vi "PID_controller_02.vi"() -> ()   [LabVIEW 2011]
uses:
  <vilib>/Platform/TimedLoop/XDataNode/nitl_modes.ctl
  <vilib>/Platform/TimedLoop/XDataNode/timing_clust.ctl
  <vilib>/Platform/TimedLoop/XDataNode/wakeup.ctl
  <vilib>/Platform/TimedLoop/XDataNode/XDataNode.xnode
  <vilib>/Platform/TimedLoop/XDataNode/XDNodeRunTimeDep.lvlib
panel:
  out "tan(angle)":dbl
  in  "stop":bool
  out "duration (s)":dbl
  in  "Period (s)":dbl
  out "Process value":dbl
  out "prev error":dbl
  out "derivative":dbl
  out "integral":dbl
  out "error":dbl
  out "Current angle (deg)":dbl
  in  "Kd":dbl
  in  "Ki":dbl
  in  "Kp":dbl
  out "Current value (torr)":dbl
  in  "Set Point (torr)":dbl
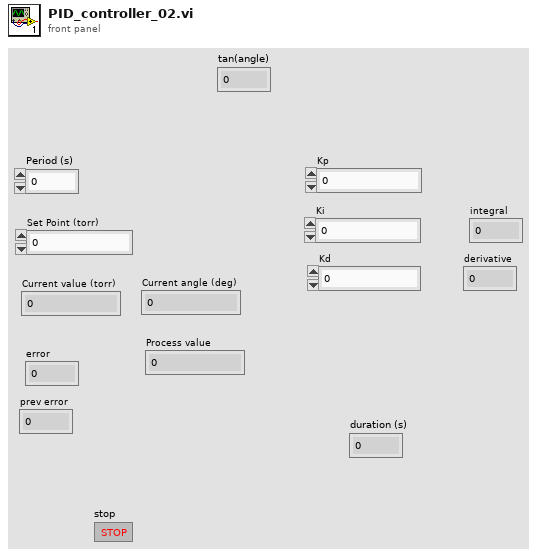
[diagram p1: front panel]
types:
  T1 = typedef "XDNodeRunTimeDep.lvlib/nitl_modes.ctl" = enum32{"No Change", "Process missed periods, maintain original phase", "Discard missed periods, maintain original phase", "Process missed periods, ignore original phase", "Discard missed periods, ignore original phase"}
  T2 = typedef "XDNodeRunTimeDep.lvlib/timing_clust.ctl" = cluster{"Expected End [f-1]":u64, "Actual End [f-1]":u64, "Finished Late? [f-1]":bool, "Expected End [i-1]":u64, "Actual End [i-1]":u64, "Finished Late? [i-1]":bool, "Expected Start [i]":u64, "Actual Start [i]":u64, "Expected Start [f]":u64, "Actual Start [f]":u64, "Source Name":string, "Structure Name":string, "Period":i64, "Deadline":i64, "Offset":i64, "Start":i64, "Priority":i32, "Timeout":i32, "Mode":T1, "Wakeup Reason":T3, "Error":errorcluster, "Source Type":string, "Secondary Source Type":string, "Global End Time":u64, "Global Start Time":u64, "Frame Duration":u64, "Iteration Duration":u64, "Assigned CPU":i32, "I/O Scan Engine Mode":u32}
  T3 = typedef "XDNodeRunTimeDep.lvlib/wakeup.ctl" = enum32{"Normal", "Aborted", "Asynchronous wakeup", "Timing source error", "Timed loop error", "Timeout"}
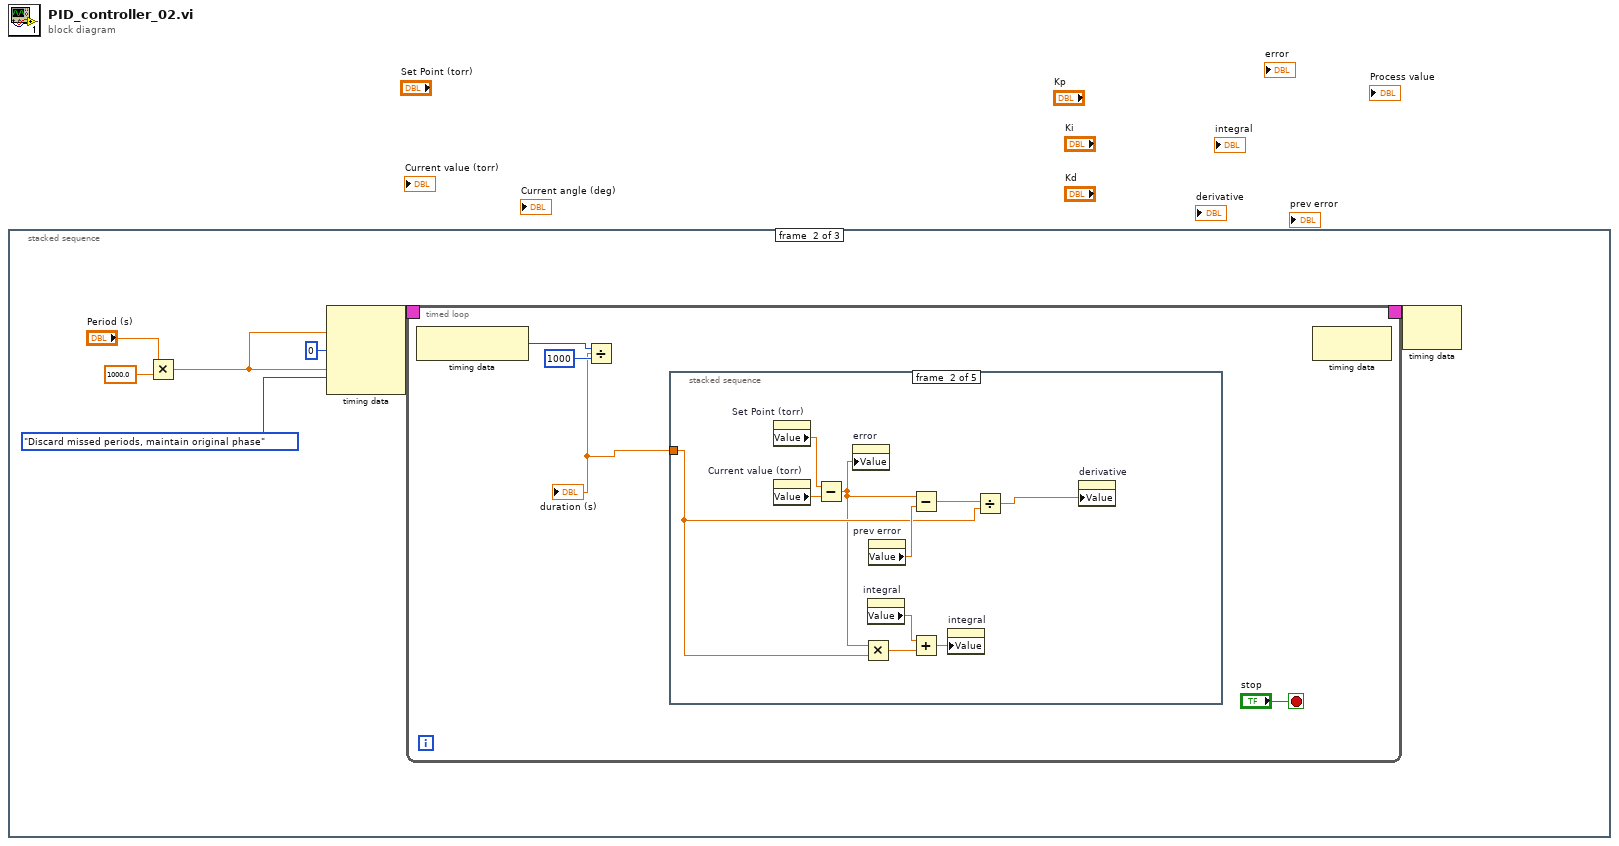
[diagram p0: block diagram]
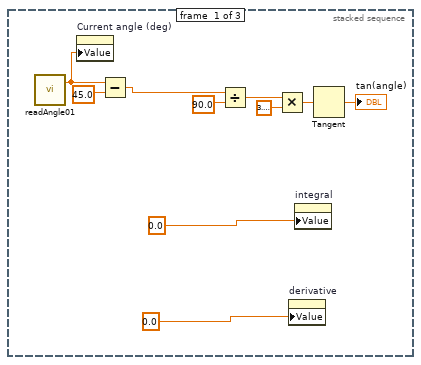
[diagram p2: hidden frame]
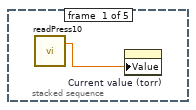
[diagram p3: hidden frame]
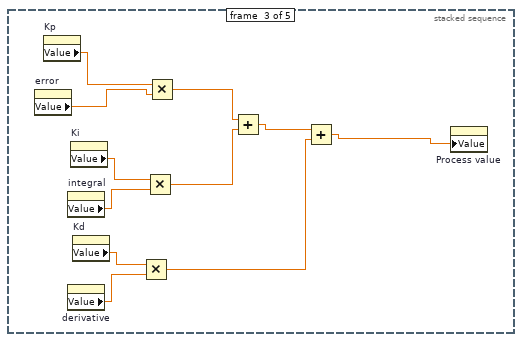
[diagram p4: hidden frame]
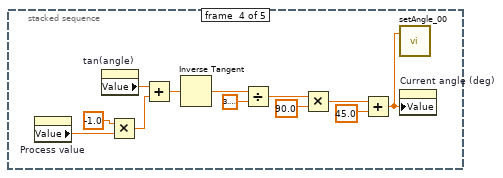
[diagram p5: hidden frame]
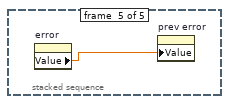
[diagram p6: hidden frame]
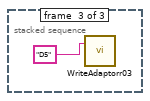
[diagram p7: hidden frame]
diagram:
  n1 = stacked-sequence {
    frame #0 {
      n2 = call "readAngle01.vi"() -> ("angle"=w7:dbl)  [unwired: 1 in, 1 out]
      n3 = property on="Current angle (deg)" class="DigNum (strict)"("Value"=w7) -> ()  [unwired: 2 in, 2 out]
      n4 = Subtract(x=w7, y=45.0) -> (x-y=w1:dbl)
      n5 = Divide(x=w1, y=90.0) -> (x/y=w5:dbl)
      n6 = Multiply(x=w5, y=3.141592653589793) -> (x*y=w3:dbl)
      n7 = property on="derivative" class="DigNum (strict)"("Value"=0.0 ("derivative")) -> ()  [unwired: 2 in, 2 out]
      n8 = property on="integral" class="DigNum (strict)"("Value"=0.0 ("integral")) -> ()  [unwired: 2 in, 2 out]
      n9 = Tangent(1:w3) -> (0:→"tan(angle)":dbl)
    }
    frame #1 {
      n10 = Multiply(x="Period (s)", y=1000.0) -> (x*y=w12:dbl)
      n11 = node-c288(w12, i64 0 ("Offset"), w12, nitl_modes."Discard missed periods, maintain original phase" ("Mode")) -> (w17:T2)
      n12 = timed-loop {
        timing: w17 -> [_]
        timing-out: [_] -> w16
        stop <- "stop" stop-if-true
        n13 = node-c288() -> (w21:i64)  [unwired: 1 in]
        n14 = Divide(x=w21, y=i64 1000) -> (x/y=w19:dbl)
        "duration (s)" <- w19
        n15 = stacked-sequence {
          tunnel: w19 -> [_ w26 _ _ _]
          frame #0 {
            n16 = call "readPress10.vi"() -> ("P"=w22:dbl)  [unwired: 1 in, 1 out]
            n17 = property on="Current value (torr)" class="DigNum (strict)"("Value"=w22) -> ()  [unwired: 2 in, 2 out]
          }
          frame #1 {
            n18 = property on="Set Point (torr)" class="DigNum (strict)"() -> ("Value"=w28:dbl)  [unwired: 2 in, 2 out]
            n19 = property on="Current value (torr)" class="DigNum (strict)"() -> ("Value"=w29:dbl)  [unwired: 2 in, 2 out]
            n20 = Subtract(x=w28, y=w29) -> (x-y=w23:dbl)
            n21 = property on="error" class="DigNum (strict)"("Value"=w23) -> ()  [unwired: 2 in, 2 out]
            n22 = Multiply(x=w23, y=w26) -> (x*y=w27:dbl)
            n23 = property on="integral" class="DigNum (strict)"() -> ("Value"=w32:dbl)  [unwired: 2 in, 2 out]
            n24 = property on="prev error" class="DigNum (strict)"() -> ("Value"=w30:dbl)  [unwired: 2 in, 2 out]
            n25 = Subtract(x=w23, y=w30) -> (x-y=w25:dbl)
            n26 = Add(x=w32, y=w27) -> (x+y=w31:dbl)
            n27 = property on="integral" class="DigNum (strict)"("Value"=w31) -> ()  [unwired: 2 in, 2 out]
            n28 = Divide(x=w25, y=w26) -> (x/y=w24:dbl)
            n29 = property on="derivative" class="DigNum (strict)"("Value"=w24) -> ()  [unwired: 2 in, 2 out]
          }
          frame #2 {
            n30 = property on="error" class="DigNum (strict)"() -> ("Value"=w43:dbl)  [unwired: 2 in, 2 out]
            n31 = property on="Kp" class="DigNum (strict)"() -> ("Value"=w42:dbl)  [unwired: 2 in, 2 out]
            n32 = property on="integral" class="DigNum (strict)"() -> ("Value"=w40:dbl)  [unwired: 2 in, 2 out]
            n33 = property on="derivative" class="DigNum (strict)"() -> ("Value"=w38:dbl)  [unwired: 2 in, 2 out]
            n34 = property on="Ki" class="DigNum (strict)"() -> ("Value"=w41:dbl)  [unwired: 2 in, 2 out]
            n35 = property on="Kd" class="DigNum (strict)"() -> ("Value"=w39:dbl)  [unwired: 2 in, 2 out]
            n36 = Multiply(x=w39, y=w38) -> (x*y=w35:dbl)
            n37 = Multiply(x=w41, y=w40) -> (x*y=w36:dbl)
            n38 = Multiply(x=w42, y=w43) -> (x*y=w37:dbl)
            n39 = Add(x=w37, y=w36) -> (x+y=w34:dbl)
            n40 = Add(x=w34, y=w35) -> (x+y=w33:dbl)
            n41 = property on="Process value" class="DigNum (strict)"("Value"=w33) -> ()  [unwired: 2 in, 2 out]
          }
          frame #3 {
            n42 = property on="Process value" class="DigNum (strict)"() -> ("Value"=w53:dbl)  [unwired: 2 in, 2 out]
            n43 = property on="tan(angle)" class="DigNum (strict)"() -> ("Value"=w46:dbl)  [unwired: 2 in, 2 out]
            n44 = Multiply(x=-1.0, y=w53) -> (x*y=w54:dbl)
            n45 = Add(x=w46, y=w54) -> (x+y=w45:dbl)
            n46 = Inverse Tangent(1:w45) -> (0:w52:dbl)
            n47 = Divide(x=w52, y=3.141592653589793) -> (x/y=w50:dbl)
            n48 = Multiply(x=w50, y=90.0) -> (x*y=w48:dbl)
            n49 = Add(x=w48, y=45.0) -> (x+y=w44:dbl)
            n50 = call "setAngle_00.vi"("Angle (deg)"=w44) -> ()  [unwired: 1 in, 1 out]
            n51 = property on="Current angle (deg)" class="DigNum (strict)"("Value"=w44) -> ()  [unwired: 2 in, 2 out]
          }
          frame #4 {
            n52 = property on="error" class="DigNum (strict)"() -> ("Value"=w56:dbl)  [unwired: 2 in, 2 out]
            n53 = property on="prev error" class="DigNum (strict)"("Value"=w56) -> ()  [unwired: 2 in, 2 out]
          }
        }
        n54 = node-c288() -> ()  [unwired: 1 in, 1 out]
      }
      n55 = node-c288(w16) -> ()  [unwired: 1 out]
    }
    frame #2 {
      n56 = call "WriteAdaptorr03.vi"("string to write"="D5") -> ()  [unwired: 1 in, 1 out]
    }
  }
